vi "grSim_Robot_Command Encoder.vi"(8 "error in (no error)":errorcluster, 10 "robot":T1, 11 "Communication in":refnum<class "Communication.lvclass">) -> (0 "error out":errorcluster, 1 "Array out":u8[](array[numeric]), 3 "Communication out":refnum<class "Communication.lvclass">)   [LabVIEW 2022 SP3, in "Communication.lvclass"]
uses:
  Communication.lvclass
  Paths/Convert AI Robot to Robot Command Folder/grSim/grSim Robot Command.ctl
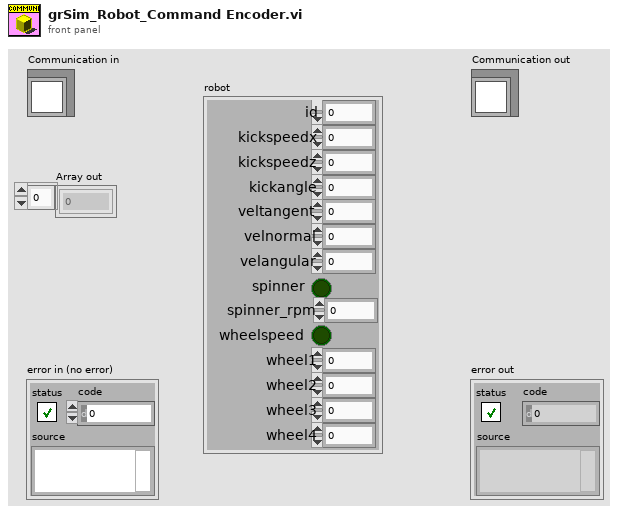
[diagram p1: front panel]
types:
  T1 = typedef "grSim Robot Command.ctl" = cluster{"id":u32, "kickspeedx":sgl, "kickspeedz":sgl, "veltangent":sgl, "velnormal":sgl, "velangular":sgl, "spinner":bool, "wheelspeed":bool, "wheel1":sgl, "wheel2":sgl, "wheel3":sgl, "wheel4":sgl, "kickangle":sgl, "spinner_rpm":sgl}
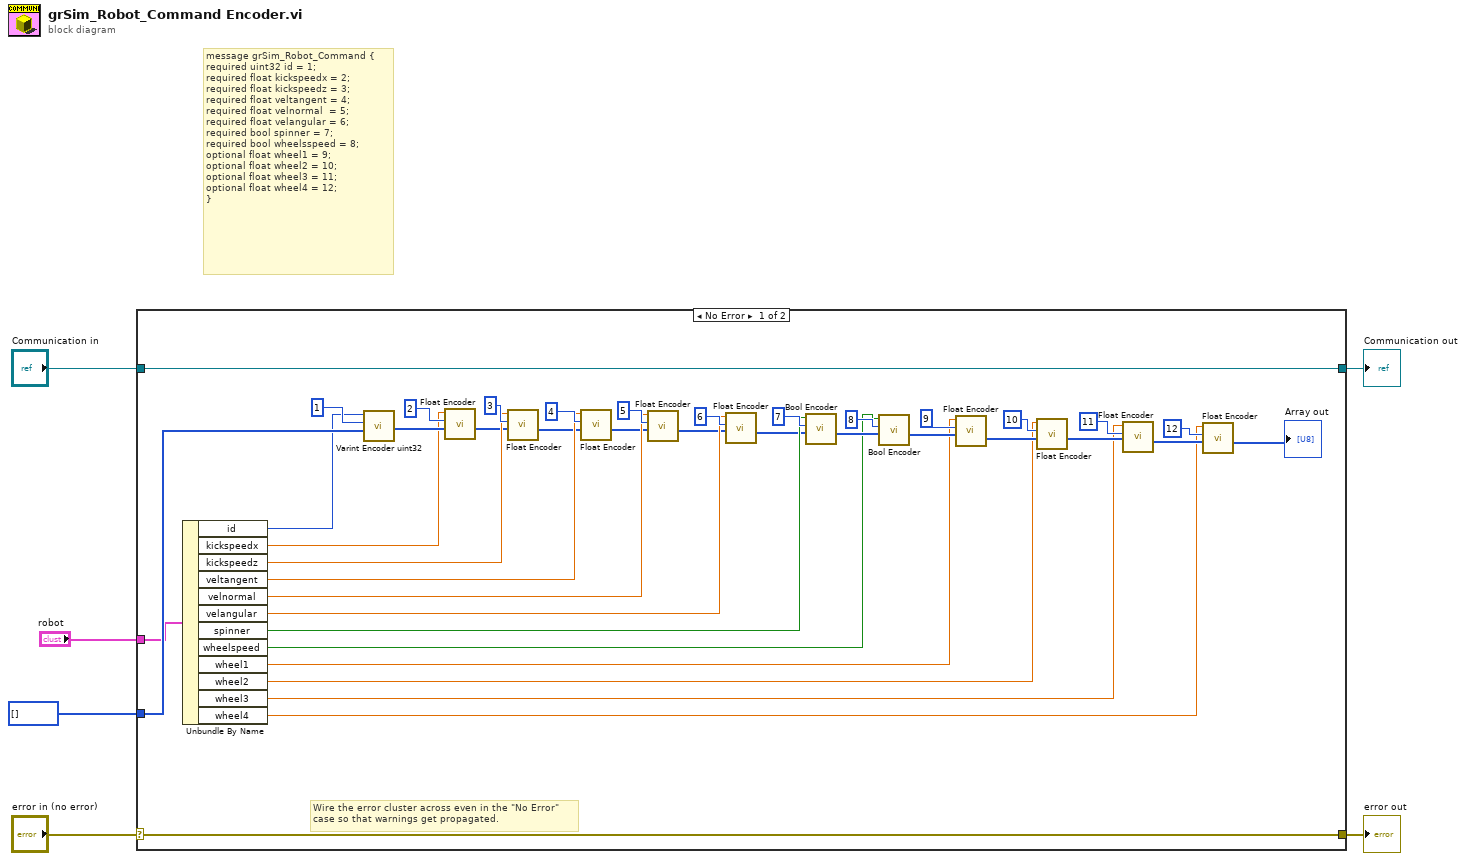
[diagram p0: block diagram]
diagram:
  # "message grSim_Robot_Command {\nrequired uint32 id = 1;\nrequired float kickspeedx = 2;\nrequired float kickspeedz = 3;\nrequired float veltangent = 4;\nrequired float velnormal  = 5;\nrequired float velangular = 6;\nrequired bool spinner = 7;\nrequired bool wheelsspeed = 8;\noptional float wheel1 = 9;\noptional float wheel2 = 10;\noptional float wheel3 = 11;\noptional float wheel4 = 12;\n}"
  n1 = case shown="No Error" "error in (no error)" {
    selector: "error in (no error)" -> [w45 w48]
    tunnel: [w45 w48] -> w5
    tunnel: [w46 w47] -> w3
    tunnel: "Communication in" -> [w46 w47]
    tunnel: u8[] [] ("Array in") -> [w43 _]
    tunnel: "robot" -> [w42 _]
    frame No Error {
      # "Wire the error cluster across even in the \"No Error\"\ncase so that warnings get propagated."
      n2 = Unbundle By Name(w42) -> ("id"=w41:u32, "kickspeedx"=w38:sgl, "kickspeedz"=w28:sgl, "veltangent"=w27:sgl, "velnormal"=w26:sgl, "velangular"=w25:sgl, "spinner"=w24:bool, "wheelspeed"=w13:bool, "wheel1"=w12:sgl, "wheel2"=w11:sgl, "wheel3"=w8:sgl, "wheel4"=w10:sgl)
      n3 = call "Varint Encoder uint32.vi"("Array In"=w43, "Key"=u32 1, "Value"=w41) -> ("Array"=w40:u8[])  [unwired: 8 in]
      n4 = call "Float Encoder.vi"("Array In"=w40, "Key"=u32 2, "Value"=w38) -> ("Array"=w23:u8[])  [unwired: 8 in]
      n5 = call "Float Encoder.vi"("Array In"=w23, "Key"=u32 3, "Value"=w28) -> ("Array"=w22:u8[])  [unwired: 8 in]
      n6 = call "Float Encoder.vi"("Array In"=w22, "Key"=u32 4, "Value"=w27) -> ("Array"=w21:u8[])  [unwired: 8 in]
      n7 = call "Float Encoder.vi"("Array In"=w21, "Key"=u32 5, "Value"=w26) -> ("Array"=w20:u8[])  [unwired: 8 in]
      n8 = call "Float Encoder.vi"("Array In"=w20, "Key"=u32 6, "Value"=w25) -> ("Array"=w19:u8[])  [unwired: 8 in]
      n9 = call "Bool Encoder.vi"("Array In"=w19, "Key"=u32 7, "Value"=w24) -> ("Array"=w18:u8[])  [unwired: 8 in]
      n10 = call "Bool Encoder.vi"("Array In"=w18, "Key"=u32 8, "Value"=w13) -> ("Array"=w17:u8[])  [unwired: 8 in]
      n11 = call "Float Encoder.vi"("Array In"=w17, "Key"=u32 9, "Value"=w12) -> ("Array"=w16:u8[])  [unwired: 8 in]
      n12 = call "Float Encoder.vi"("Array In"=w16, "Key"=u32 10, "Value"=w11) -> ("Array"=w15:u8[])  [unwired: 8 in]
      n13 = call "Float Encoder.vi"("Array In"=w15, "Key"=u32 11, "Value"=w8) -> ("Array"=w14:u8[])  [unwired: 8 in]
      n14 = call "Float Encoder.vi"("Array In"=w14, "Key"=u32 12, "Value"=w10) -> ("Array"=→"Array out":u8[])  [unwired: 8 in]
    }
    frame Error {
    }
  }
  "error out" <- w5
  "Communication out" <- w3
